vi "Get Blank Time.vi"(8 "error in (no error)":errorcluster, 11 "Neph in":refnum<class "Nephelometer.lvclass">) -> (0 "error out":errorcluster, 2 "STB":u16, 3 "Neph out":refnum<class "Nephelometer.lvclass">)   [LabVIEW 2014, in "Nephelometer.lvclass"]
uses:
  Nephelometer.lvclass
  Nephelometer.lvclass/Nephelometer.ctl
  Reusable/Session APIs/Serial/Public/Get Data/Get Long Integer.vi
  Reusable/Session APIs/Text Communication/Text Device Session.lvclass
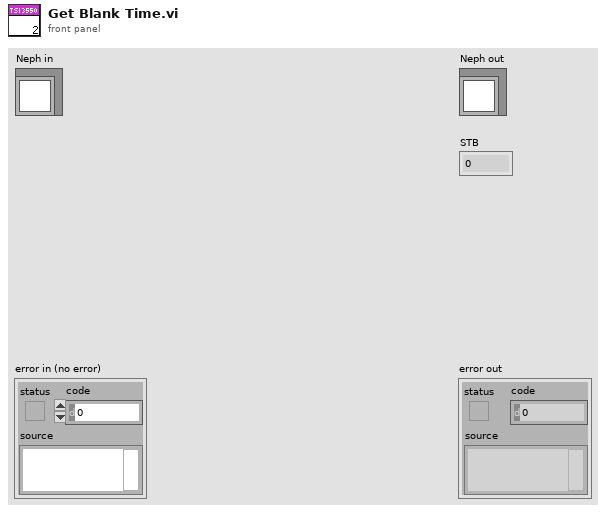
[diagram p1: front panel]
types:
  T1 = typedef "Session - Root.lvclass/Session Handle.ctl" = refnum<data-value>
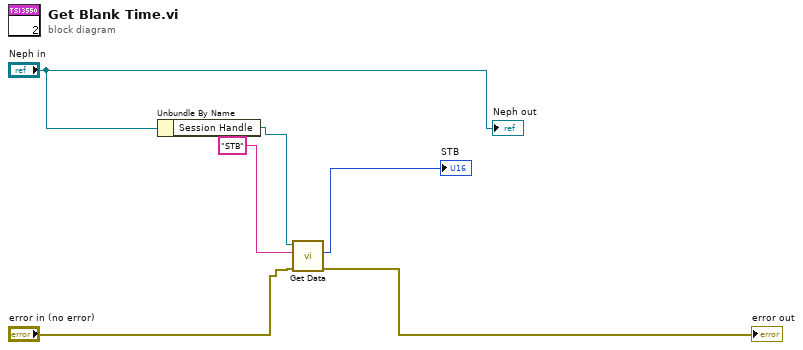
[diagram p0: block diagram]
diagram:
  n1 = Unbundle By Name("Neph in") -> ("Session Handle"=w4:T1)
  n2 = call-poly "Get Data.vi"("error in"="error in (no error)", "CMD"="STB", "handle in"=w4) -> ("error out"=→"error out":errorcluster, "DataOut"=→"STB":i32)  [unwired: 6 in, 1 out]
  "Neph out" <- "Neph in"
